vi "Set Pane Origin.vi"(8 "error in":errorcluster, 10 "Pane Origin":T1[](array[typedef]), 11 "VI Ref":refnum<vi>) -> (0 "error out":errorcluster, 3 "VI Ref":refnum<vi>)   [LabVIEW 2014]
uses:
  <vilib>/Utility/miscctls.llb/LVPointTypeDef.ctl
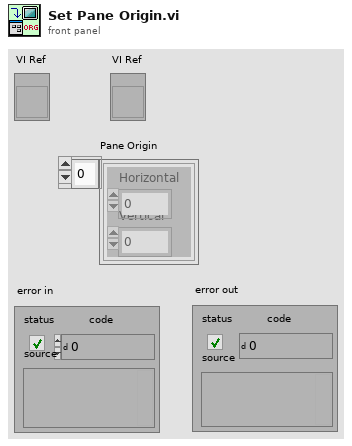
[diagram p1: front panel]
types:
  T1 = typedef "LVPointTypeDef.ctl" = cluster{"Horizontal":i16, "Vertical":i16}
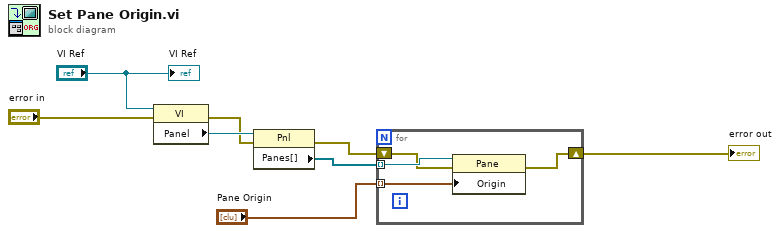
[diagram p0: block diagram]
diagram:
  n1 = property class="VI"(reference="VI Ref", error in="error in") -> (error out=w4:errorcluster, "Panel"=w7:refnum<vi>)  [unwired: 1 out]
  n2 = property class="Pnl"(reference=w7, error in=w4) -> (error out=w5:errorcluster, "Panes[]"=w6:refnum<vi>[])  [unwired: 1 out]
  n3 = for {
    tunnel: w6 -> [w12] mode=indexing
    shift-right: [w10] -> w3
    shift-left: w5 -> [w11]
    tunnel: "Pane Origin" -> [w9] mode=indexing
    n4 = property class="Pane"(reference=w12, error in=w11, "Origin"=w9) -> (error out=w10:errorcluster)  [unwired: 1 out]
  }
  "error out" <- w3
  "VI Ref" <- "VI Ref"
